vi "MGCC_FntStaMach_Initial_function.vi"   [LabVIEW 2016]
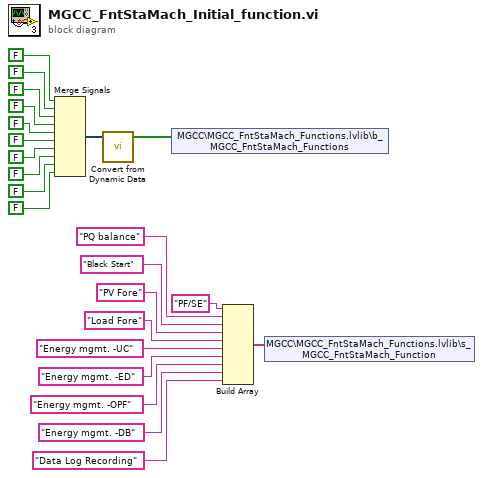
[diagram p0: block diagram]
diagram:
  n1 = Merge Signals(FALSE ("State3"), FALSE ("State3"), FALSE ("State3"), FALSE ("State3"), FALSE ("State3"), FALSE ("State3"), FALSE ("State3"), FALSE ("State3"), FALSE ("State3"), FALSE ("State3")) -> (w13:dynamicdata)
  n2 = call "Convert from Dynamic Data"("Dynamic Data Type"=w13) -> ("Array"=w1:bool[])  [unwired: 3 in]
  n3 = shared-variable "MGCC\\MGCC_FntStaMach_Functions.lvlib\\b_MGCC_FntStaMach_Functions"(w1) -> ()  [unwired: 1 in, 1 out]
  n4 = Build Array("PF/SE", "PQ balance", "Black Start", "PV Fore", "Load Fore", "Energy mgmt. -UC", "Energy mgmt. -ED", "Energy mgmt. -OPF", "Energy mgmt. -DB", "Data Log Recording") -> (w2:string[])
  n5 = shared-variable "MGCC\\MGCC_FntStaMach_Functions.lvlib\\s_MGCC_FntStaMach_Function"(w2) -> ()  [unwired: 1 in, 1 out]
